vi "paint_targets.vi"(10 "XYGraph Refnum":refnum<vi>) -> ()   [LabVIEW 2011]
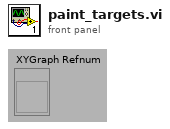
[diagram p1: front panel]
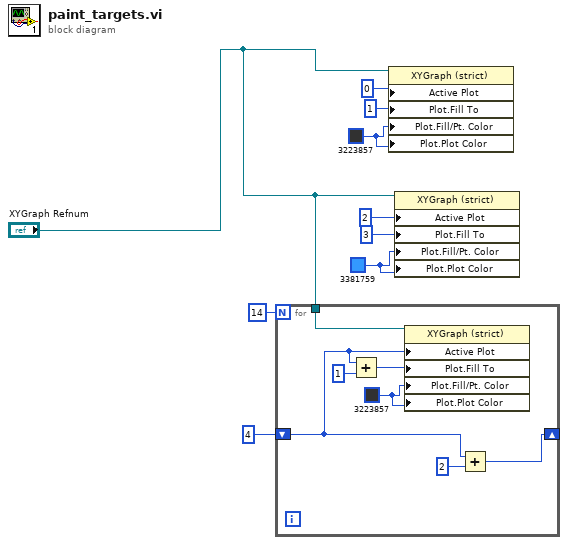
[diagram p0: block diagram]
diagram:
  w9 = u32 3381759
  w8 = u32 3223857
  n1 = for {
    N: 14 -> [_]
    shift-right: [w15] -> _
    shift-left: i16 4 ("Plot.Fill To") -> [w11]
    tunnel: "XYGraph Refnum" -> [w10]
    w14 = u32 3223857
    n2 = Add(x=w11, y=1) -> (x+y=w13:i32)
    n3 = property on="Property Node" class="XYGraph (strict)"(reference=w10, "Active Plot"=w11, "Plot.Fill To"=w13, "Plot.Fill/Pt. Color"=w14, "Plot.Plot Color"=w14) -> ()  [unwired: 1 in, 2 out]
    n4 = Add(x=w11, y=i16 2) -> (x+y=w15:i16)
  }
  n5 = property on="Property Node" class="XYGraph (strict)"(reference="XYGraph Refnum", "Active Plot"=u32 0, "Plot.Fill To"=i16 1, "Plot.Fill/Pt. Color"=w8, "Plot.Plot Color"=w8) -> ()  [unwired: 1 in, 2 out]
  n6 = property on="Property Node" class="XYGraph (strict)"(reference="XYGraph Refnum", "Active Plot"=u32 2, "Plot.Fill To"=i16 3, "Plot.Fill/Pt. Color"=w9, "Plot.Plot Color"=w9) -> ()  [unwired: 1 in, 2 out]
